vi "Service map insert.vi"(4 "error in (no error)":errorcluster, 6 "Map entry":T1={"CobID"=0, "Data offset"=4, "Data size"=4, "Destination"=refnum}, 7 "CANopen in":refnum<class "CANopen.lvclass">) -> (0 "error out":errorcluster, 3 "CANopen out":refnum<class "CANopen.lvclass">)   [LabVIEW 2017, in "canopen.lvlib" / "CANopen.lvclass"]
doc: "Appends a new entry inside the service map. The insertion is protected by a mutex in order to prevent race conditions with \"Service map delete\"."
uses:
  CANopen.lvclass
  CANopen.lvclass/CANopen.ctl
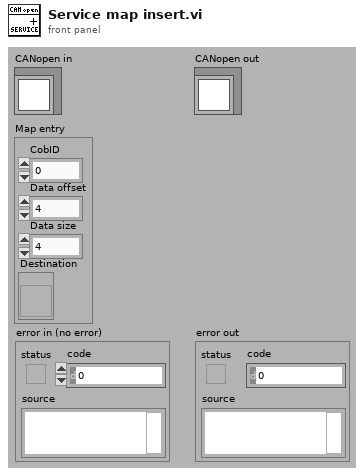
[diagram p1: front panel]
types:
  T1 = cluster{"CobID":u32, "Data offset":u8, "Data size":u8, "Destination":refnum<vi>}
  T2 = typedef "Semaphore RefNum" = refnum<k1>
  T3 = cluster{"CobID":u32, "Data offset":u8, "Data size":u8, "Destination":refnum<vi>}[]
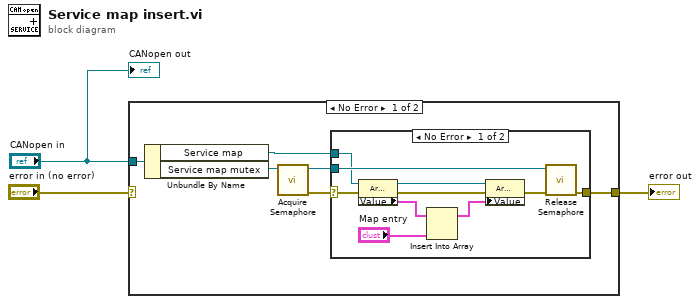
[diagram p0: block diagram]
diagram:
  n1 = case shown="No Error" "error in (no error)" {
    selector: "error in (no error)" -> [_ w21]
    tunnel: [w9 w21] -> w3
    tunnel: "CANopen in" -> [w5 _]
    frame No Error {
      n2 = Unbundle By Name(w5) -> ("Service map"=w6:refnum<vi>, "Service map mutex"=w7:T2)
      n3 = call <vilib>:"Acquire Semaphore.vi"("semaphore"=w7) -> ("error out"=w4:errorcluster, "semaphore out"=w8:T2)  [unwired: 2 in, 3 out]
      n4 = case shown="No Error" w4 {
        selector: w4 -> [w10 w20]
        tunnel: [w19 w20] -> w9
        tunnel: w8 -> [w14 _]
        tunnel: w6 -> [w13 _]
        frame No Error {
          n5 = property class="Arr (strict)"(reference=w13, error in=w10) -> (reference out=w12:refnum<vi>, error out=w15:errorcluster, "Value"=w16:T3)
          n6 = Insert Into Array(array=w16, new element="Map entry") -> (w18:T3)  [unwired: 1 in]
          n7 = property class="Arr (strict)"(reference=w12, error in=w15, "Value"=w18) -> (error out=w17:errorcluster)  [unwired: 1 out]
          n8 = call <vilib>:"Release Semaphore.vi"("error in (no error)"=w17, "semaphore"=w14) -> ("error out"=w19:errorcluster)  [unwired: 5 out]
        }
        frame Error {
        }
      }
    }
    frame Error {
    }
  }
  "error out" <- w3
  "CANopen out" <- "CANopen in"
